vi "table 1.vi"() -> ()   [LabVIEW 2019]
panel:
  out "Array 2":dbl[](array[numeric])
  in  "dimension":i32
  in  "element":dbl
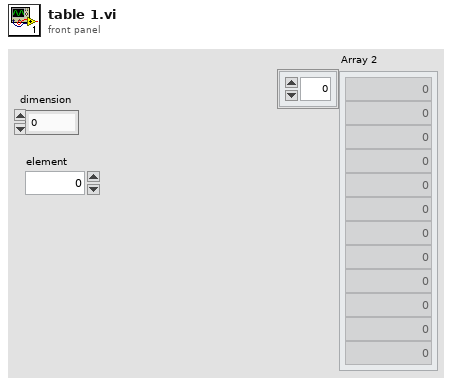
[diagram p1: front panel]
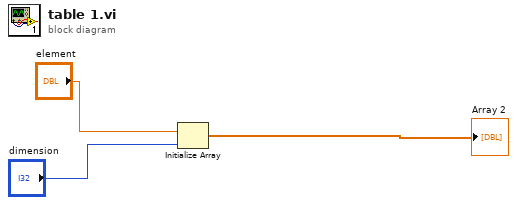
[diagram p0: block diagram]
diagram:
  n1 = Initialize Array("element", "dimension") -> (→"Array 2":dbl[])
